vi "4-Byte-to-Byte-Array.vi"(7 "4 Byte in":u32=1091567616 format="%032b") -> (3 "Byte array out":u8[](array[numeric]) format="%08b")   [LabVIEW 2019]
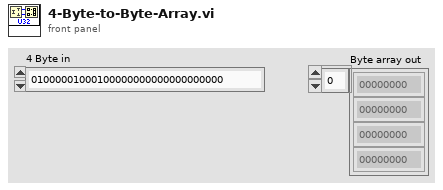
[diagram p1: front panel]
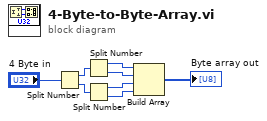
[diagram p0: block diagram]
diagram:
  n1 = Split Number(x="4 Byte in") -> (hi(x)=w2:u16, lo(x)=w3:u16)
  n2 = Split Number(x=w2) -> (hi(x)=w1:u8, lo(x)=w6:u8)
  n3 = Split Number(x=w3) -> (hi(x)=w5:u8, lo(x)=w4:u8)
  n4 = Build Array(w1, w6, w5, w4) -> (→"Byte array out":u8[])
